vi "AdjustVINameAndPath.vi"(8 "OldVIPath":path, 9 "NewVIPath":path, 10 "OldVIName":string, 11 "NewVIName":string) -> (0 "RelativePath":bool, 1 "VIPath":path, 3 "VINameOut":string)   [LabVIEW 2016, in "VINode.lvclass"]
uses:
  <resource>/Framework/Providers/Open_GDS/UML/VINode_class/VINode.lvclass
  <resource>/Framework/Providers/Open_GDS/UML/UMLEditor/UMLEditor_StoredPathes.ctl
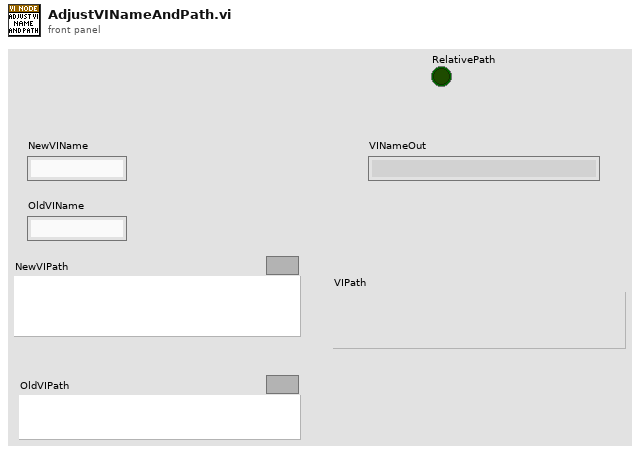
[diagram p1: front panel]
types:
  T1 = typedef "UMLEditor_StoredPathes.ctl" = enum16{"LastSearchPath", "QueuedArrayStateVI", "ClassBasePath", "ViTemplatePath", "ApplicationTemplatePath", "IniFilePath", "WizDir", "RevPlugInPath"}
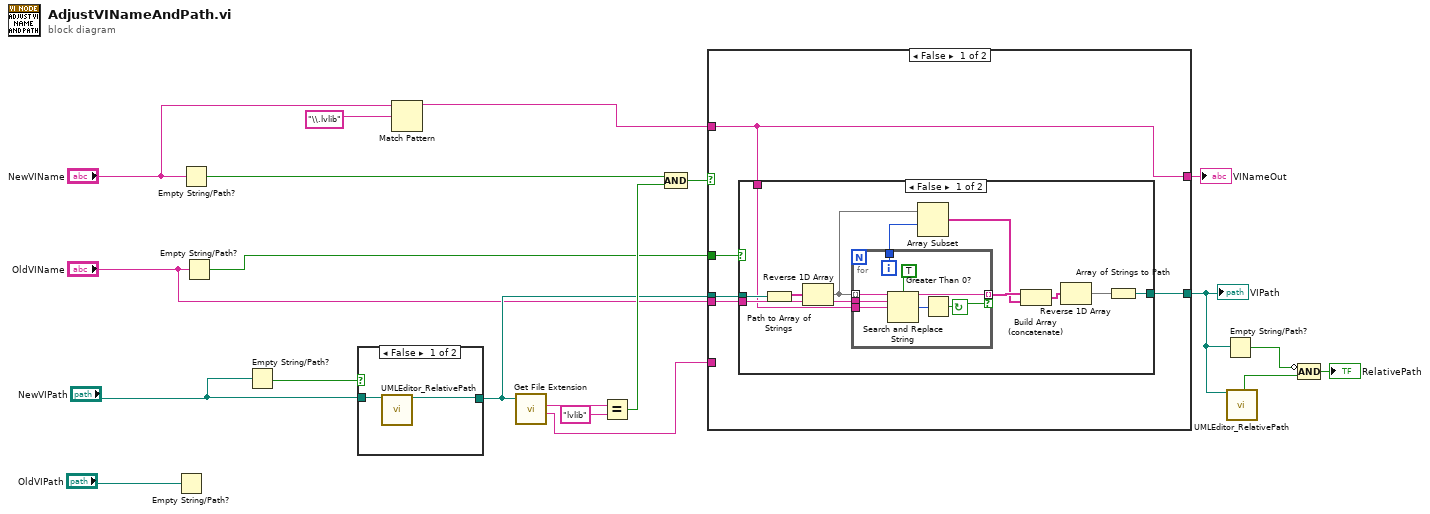
[diagram p0: block diagram]
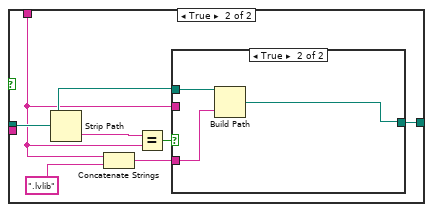
[diagram p2: hidden frame]
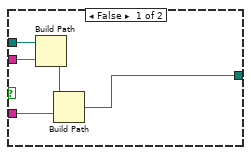
[diagram p3: hidden frame]
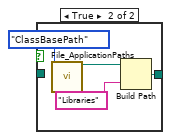
[diagram p5: hidden frame]
diagram:
  n1 = Empty String/Path?(string/path="OldVIPath") -> ()  [unwired: 1 out]
  n2 = Empty String/Path?(string/path="NewVIName") -> (empty?=w5:bool)
  n3 = Empty String/Path?(string/path="OldVIName") -> (empty?=w8:bool)
  n4 = Empty String/Path?(string/path="NewVIPath") -> (empty?=w15:bool)
  n5 = case shown="False" w15 {
    tunnel: "NewVIPath" -> [w22 _]
    tunnel: [w21 w23] -> w7
    frame False {
      n6 = call <resource>:"UMLEditor_RelativePath.vi"("Path In"=w22) -> ("ConvertToAbsolutePath(If possible)"=w21:path)  [unwired: 1 in, 17 out]
    }
    frame True {
      n7 = call <resource>:"File_ApplicationPaths.vi"("PathName"=UMLEditor_StoredPathes."ClassBasePath" ("UMLPathes")) -> ("Path Out"=w25:path)  [unwired: 3 in, 15 out]
      n8 = Build Path(base path=w25, name or relative path="Libraries") -> (appended path=w23:path)
    }
  }
  n9 = Match Pattern(string="NewVIName", regular expression="\\.lvlib") -> (before substring=w4:string)  [unwired: 4 out]
  n10 = call <vilib>:"Get File Extension.vi"("file"=w7) -> ("filename without extension"=w9:string, "lowercase file extension"=w14:string)  [unwired: 6 in, 3 out]
  n11 = Equal?(x=w14, y="lvlib") -> (x = y?=w12:bool)
  n12 = Compound Arithmetic op=AND(w5, w12) -> (w11:bool)
  n13 = case shown="False" w11 {
    tunnel: [w28 w67] -> w10
    tunnel: w9 -> [_ w67]
    tunnel: w4 -> [w28 _]
    tunnel: w8 -> [w31 _]
    tunnel: w7 -> [w30 w66]
    tunnel: "OldVIName" -> [w29 _]
    tunnel: [w27 w66] -> w2
    frame False {
      n14 = case shown="False" w31 {
        tunnel: w30 -> [w42 w55]
        tunnel: w29 -> [w40 _]
        tunnel: w28 -> [w39 w54]
        tunnel: [w37 w51] -> w27
        frame False {
          n15 = Path to Array of Strings(0:w42) -> (2:w41:string[])  [unwired: 1 out]
          n16 = Reverse 1D Array(array=w41) -> (reversed array=w34:string[])
          n17 = for {
            tunnel: w34 -> [w50] mode=indexing
            tunnel: w40 -> [w49]
            tunnel: w39 -> [w48]
            tunnel: [w46] -> w38 mode=indexing if=w44
            tunnel: [w43] -> w33
            i -> [w43]
            stop <- w44 continue-if-true
            n18 = Search and Replace String(case sensitive?=TRUE ("ignore case? (F)"), input string=w50, search string=w49, replace string=w48) -> (result string=w46:string, number of replacements=w45:i32)  [unwired: 4 in, 2 out]
            n19 = Greater Than 0?(x=w45) -> (x > 0?=w44:bool)
          }
          n20 = Array Subset(array=w34, index=w33) -> (w32:string[])  [unwired: 1 in]
          n21 = Build Array (concatenate)(w38, w32) -> (w35:string[])
          n22 = Reverse 1D Array(array=w35) -> (reversed array=w36:string[])
          n23 = Array of Strings to Path(0:w36) -> (2:w37:path)  [unwired: 1 in]
        }
        frame True {
          n24 = Strip Path(path=w55) -> (name=w57:string)  [unwired: 1 out]
          n25 = Concatenate Strings(w54, ".lvlib" ("y")) -> (w52:string)
          n26 = Equal?(x=w57, y=w54) -> (x = y?=w56:bool)
          n27 = case shown="True" w56 {
            tunnel: w55 -> [w62 w65]
            tunnel: w54 -> [w61 _]
            tunnel: w52 -> [w59 w64]
            tunnel: [w58 w63] -> w51
            frame False {
              n28 = Build Path(base path=w62, name or relative path=w61) -> (appended path=w60:path)
              n29 = Build Path(base path=w60, name or relative path=w59) -> (appended path=w58:path)
            }
            frame True {
              n30 = Build Path(base path=w65, name or relative path=w64) -> (appended path=w63:path)
            }
          }
        }
      }
    }
    frame True {
    }
  }
  "VINameOut" <- w10
  "VIPath" <- w2
  n31 = Empty String/Path?(string/path=w2) -> (empty?=w20:bool)
  n32 = call <resource>:"UMLEditor_RelativePath.vi"("Path In"=w2) -> ("ConvertedToARelativePath"=w19:bool)  [unwired: 1 in, 17 out]
  n33 = Compound Arithmetic op=AND(invert w20, w19) -> (→"RelativePath":bool)
